vi "ingles español.vi"(0 "UI Actor in":refnum<class "UI Actor.lvclass">, 1 "Message Enquuer":refnum<class "Message Enqueuer.lvclass">, 2 "Soda?":bool, 3 "Credito":dbl, 5 "MXN?":bool, 7 "Coins Enquuer":refnum<class "Message Enqueuer.lvclass">, 9 "Products Enquuer":refnum<class "Message Enqueuer.lvclass">, 11 "Indice":i32, 12 "Producto":string, 13 "Costo":dbl, 14 "Inventario":dbl) -> (4 "UI Actor out":refnum<class "UI Actor.lvclass">)   [LabVIEW 2020, in "UI Actor.lvlib" / "UI Actor.lvclass"]
uses:
  UI Actor.lvclass
  <vilib>/ActorFramework/Message Enqueuer/Message Enqueuer.lvclass
  C:/Program Files (x86)/National Instruments/LabVIEW 2020/vi.lib/ActorFramework/Actor/Actor.lvclass
  UI Actor.lvclass/UI Actor.ctl
  <vilib>/ActorFramework/Actor/Actor.lvclass/Actor.ctl
  USD Actor Messages/Update Coins Msg/Update Coins Msg.lvclass/Update Coins Msg.ctl
  <vilib>/ActorFramework/Message Enqueuer/Message Enqueuer.lvclass/Message Enqueuer.ctl
  MXN Actor Messages/Update Coins Msg/Update Coins Msg.lvclass/Update Coins Msg.ctl
  UI Actor Messages/creditUpdate Msg/creditUpdate Msg.lvclass/creditUpdate Msg.ctl
  MSG Messages/Update MSG Msg/Update MSG Msg.lvclass/Update MSG Msg.ctl
  <vilib>/ActorFramework/Message Enqueuer/Enqueue.vi
  USD Actor Messages/Update Coins Msg/Update Coins Msg.lvclass
  C:/Program Files (x86)/National Instruments/LabVIEW 2020/vi.lib/ActorFramework/Message/Message.lvclass
  MXN Actor Messages/Update Coins Msg/Update Coins Msg.lvclass
  UI Actor Messages/creditUpdate Msg/creditUpdate Msg.lvclass
  MSG Messages/Update MSG Msg/Update MSG Msg.lvclass
  <vilib>/ActorFramework/Message Priority Queue/Priority Enqueue.vi
  <vilib>/ActorFramework/Actor/Actor.lvclass
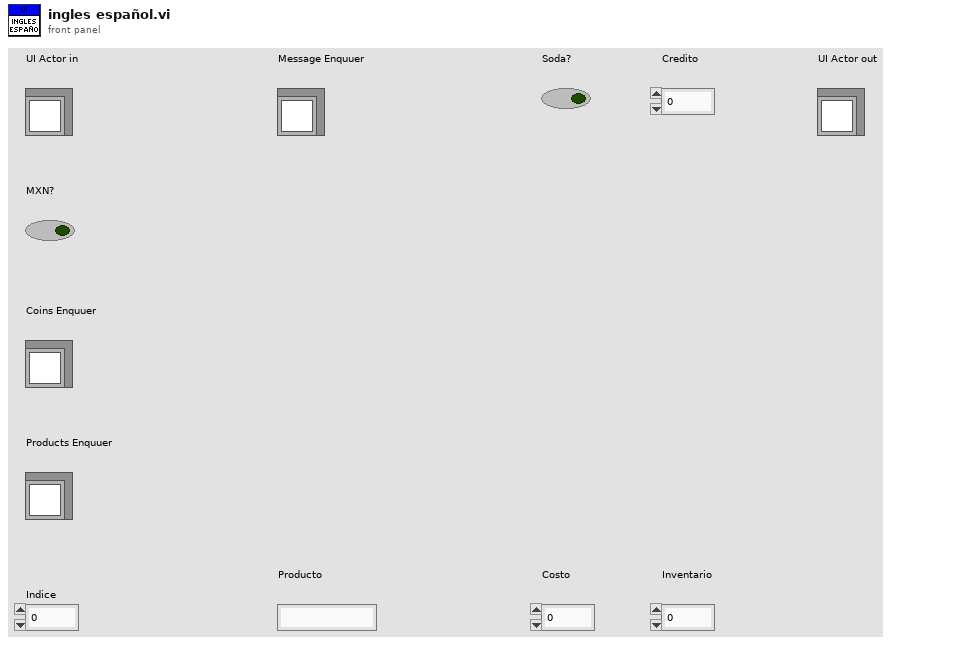
[diagram p1: front panel]
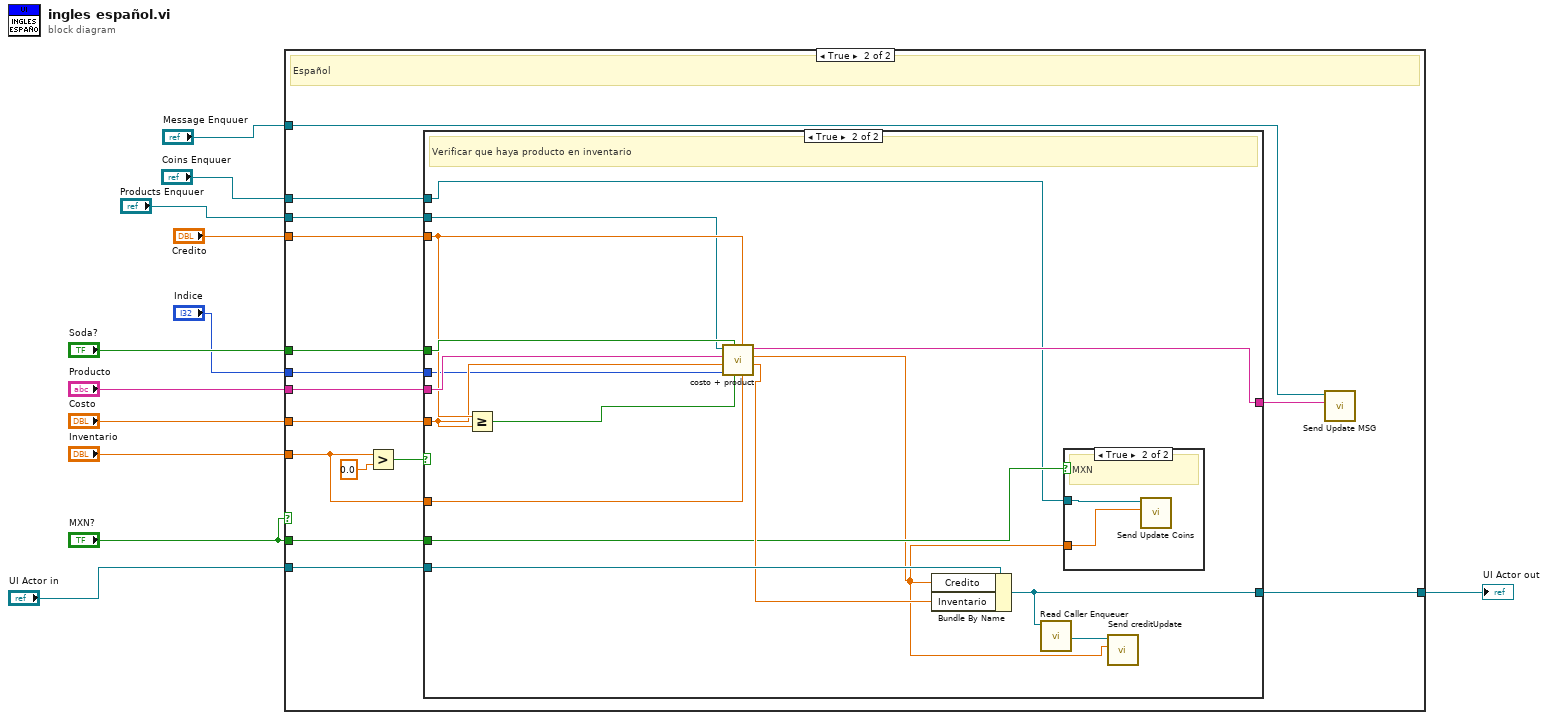
[diagram p0: block diagram]
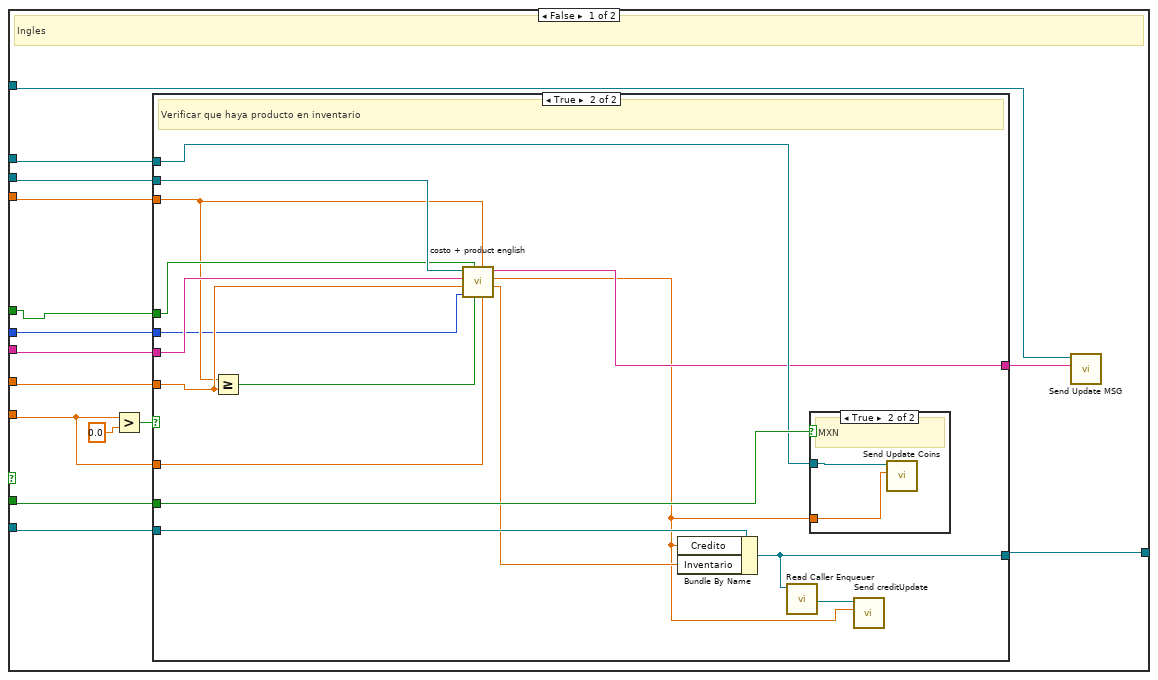
[diagram p2: hidden frame]
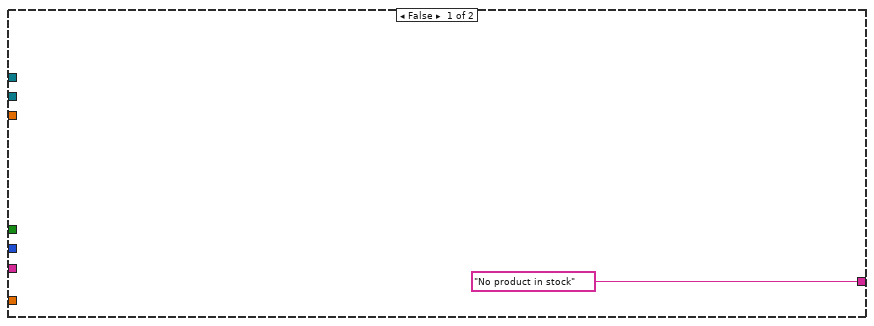
[diagram p3: hidden frame]
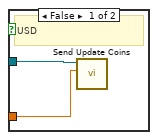
[diagram p4: hidden frame]
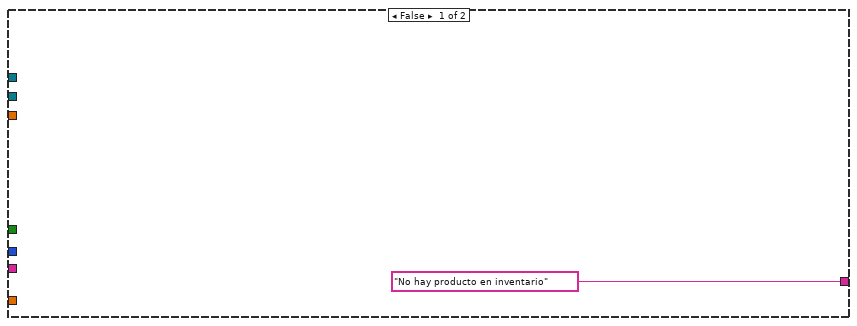
[diagram p5: hidden frame]
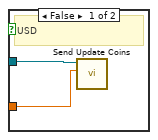
[diagram p6: hidden frame]
diagram:
  n1 = case shown="True" "MXN?" {
    tunnel: "Producto" -> [w19 w63]
    tunnel: "Soda?" -> [w20 w62]
    tunnel: "Credito" -> [w21 w61]
    tunnel: "Costo" -> [w18 w60]
    tunnel: "Message Enquuer" -> [w24 w58]
    tunnel: "UI Actor in" -> [w15 w55]
    tunnel: [w14 w54] -> w8
    tunnel: "Inventario" -> [w17 w53]
    tunnel: "Products Enquuer" -> [w22 w52]
    tunnel: "MXN?" -> [w16 w51]
    tunnel: "Coins Enquuer" -> [w23 w50]
    tunnel: "Indice" -> [w13 w49]
    frame False {
      # "Ingles"
      n2 = Greater?(x=w17, y=0.0) -> (0:w26:bool)
      n3 = case shown="True" w26 {
        tunnel: w19 -> [_ w37]
        tunnel: w20 -> [_ w36]
        tunnel: w21 -> [_ w30]
        tunnel: w18 -> [_ w35]
        tunnel: ["No product in stock" w38] -> w27
        tunnel: w15 -> [_ w44]
        tunnel: [_ w43] -> w14
        tunnel: w17 -> [_ w33]
        tunnel: w22 -> [_ w39]
        tunnel: w16 -> [_ w41]
        tunnel: w23 -> [_ w40]
        tunnel: w13 -> [_ w29]
        frame False {
        }
        frame True {
          # "Verificar que haya producto en inventario"
          n4 = Greater Or Equal?(x=w30, y=w35) -> (x >= y?=w34:bool)
          n5 = call "costo + product english.vi"("Inventario"=w33, "Credito"=w30, "Boolean"=w34, "Soda?"=w36, "Indice"=w29, "Costo"=w35, "Producto"=w37, "Message Enqueuer in"=w39) -> ("Numeric 2"=w32:dbl, "Numeric"=w31:dbl, "String"=w38:string)  [unwired: 1 in]
          n6 = Bundle By Name(cluster=w44, "Credito"=w31, "Inventario"=w32) -> (w43:refnum<class "UI Actor.lvclass">)
          n7 = call <vilib>:"Read Caller Enqueuer.vi"("Actor"=w43) -> ("Caller Enqueuer"=w42:refnum<class "Message Enqueuer.lvclass">)  [unwired: 10 in]
          n8 = case shown="True" w41 {
            tunnel: w40 -> [w46 w48]
            tunnel: w31 -> [w45 w47]
            frame False {
              # "USD"
              n9 = call "Send Update Coins.vi"("Credito Update"=w45, "Message Enqueuer"=w46) -> ()  [unwired: 8 in, 2 out]
            }
            frame True {
              # "MXN"
              n10 = call "Send Update Coins.vi"("Credito Update"=w47, "Message Enqueuer"=w48) -> ()  [unwired: 8 in, 2 out]
            }
          }
          n11 = call "Send creditUpdate.vi"("Credit"=w31, "Message Enqueuer"=w42) -> ()  [unwired: 8 in, 2 out]
        }
      }
      n12 = call "Send Update MSG.vi"("Update message"=w27, "Message Enqueuer"=w24) -> ()  [unwired: 8 in, 2 out]
    }
    frame True {
      # "Español"
      n13 = Greater?(x=w53, y=0.0) -> (0:w57:bool)
      n14 = case shown="True" w57 {
        tunnel: w63 -> [_ w80]
        tunnel: w62 -> [_ w79]
        tunnel: w61 -> [_ w77]
        tunnel: w60 -> [_ w76]
        tunnel: ["No hay producto en inventario" w75] -> w59
        tunnel: w55 -> [_ w74]
        tunnel: [_ w73] -> w54
        tunnel: w53 -> [_ w72]
        tunnel: w52 -> [_ w71]
        tunnel: w51 -> [_ w68]
        tunnel: w50 -> [_ w67]
        tunnel: w49 -> [_ w65]
        frame False {
        }
        frame True {
          # "Verificar que haya producto en inventario"
          n15 = Greater Or Equal?(x=w77, y=w76) -> (x >= y?=w78:bool)
          n16 = call "costo + product.vi"("Inventario"=w72, "Credito"=w77, "Boolean"=w78, "Soda?"=w79, "Indice"=w65, "Costo"=w76, "Producto"=w80, "Message Enqueuer in"=w71) -> ("Numeric 2"=w70:dbl, "Numeric"=w66:dbl, "String"=w75:string)  [unwired: 1 in]
          n17 = Bundle By Name(cluster=w74, "Credito"=w66, "Inventario"=w70) -> (w73:refnum<class "UI Actor.lvclass">)
          n18 = call <vilib>:"Read Caller Enqueuer.vi"("Actor"=w73) -> ("Caller Enqueuer"=w69:refnum<class "Message Enqueuer.lvclass">)  [unwired: 10 in]
          n19 = case shown="True" w68 {
            tunnel: w67 -> [w82 w84]
            tunnel: w66 -> [w81 w83]
            frame False {
              # "USD"
              n20 = call "Send Update Coins.vi"("Credito Update"=w81, "Message Enqueuer"=w82) -> ()  [unwired: 8 in, 2 out]
            }
            frame True {
              # "MXN"
              n21 = call "Send Update Coins.vi"("Credito Update"=w83, "Message Enqueuer"=w84) -> ()  [unwired: 8 in, 2 out]
            }
          }
          n22 = call "Send creditUpdate.vi"("Credit"=w66, "Message Enqueuer"=w69) -> ()  [unwired: 8 in, 2 out]
        }
      }
      n23 = call "Send Update MSG.vi"("Update message"=w59, "Message Enqueuer"=w58) -> ()  [unwired: 8 in, 2 out]
    }
  }
  "UI Actor out" <- w8
